vi "Init.vi"(8 "error in (no error)":errorcluster, 9 "Access (Read/Write)":enum16{"read/write", "read-only", "write-only"}(ring), 10 "Operation (Open or Create)":T1(ring)=enum."open or create", 11 "Path":path) -> (0 "error out":errorcluster, 3 "FileStream out":refnum<class "FileStream.lvclass">)   [LabVIEW 2020, in "Stream.lvlib" / "FileStream.lvclass"]
uses:
  FileStream.lvclass
  Stream/Stream.lvclass
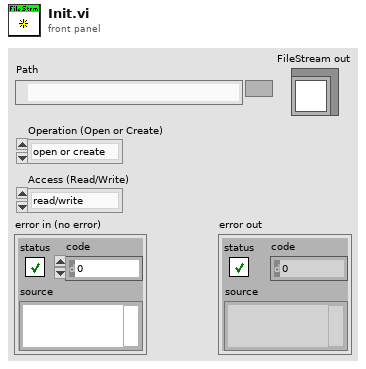
[diagram p1: front panel]
types:
  T1 = enum16{"open", "replace", "create", "open or create", "replace or create", "replace or create with confirmation"}
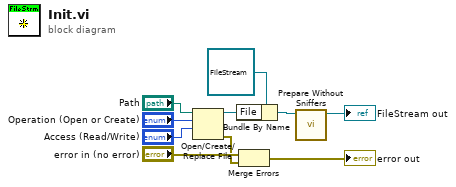
[diagram p0: block diagram]
diagram:
  n1 = Open/Create/Replace File(file path (use dialog)="Path", operation (0:open)="Operation (Open or Create)", access (0:read/write)="Access (Read/Write)") -> (refnum out=w5:refnum<file>, error out=w3:errorcluster)  [unwired: 3 in, 1 out]
  n2 = Bundle By Name(cluster=refnum<class "FileStream.lvclass"> refnum ("Stream:FileStream.lvclass"), "File"=w5) -> (w2:refnum<class "FileStream.lvclass">)
  n3 = Merge Errors("error in (no error)", w3) -> (→"error out":errorcluster)
  n4 = call "Prepare Without Sniffers.vi"("Stream in"=w2) -> ("Stream out"=→"FileStream out":refnum<class "FileStream.lvclass">)  [unwired: 9 in, 1 out]
